vi "Auton Mode Determiner.vi"() -> ()   [LabVIEW 2013]
panel:
  in  "Auton Mode":dbl
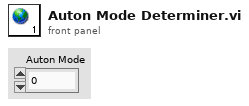
[diagram p1: front panel]
diagram:
